vi "for_v0_v1.vi"() -> ()   [LabVIEW 2009]
panel:
  out "Numeric":dbl
  in  "Delay (ms)":dbl(slide)=101.38095238095238 min=0.0 max=2000.0 step=100.0 scale=10.0..200.0
  out "Meter":dbl(knob) scale=0.0..100.0
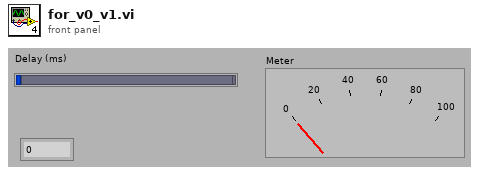
[diagram p1: front panel]
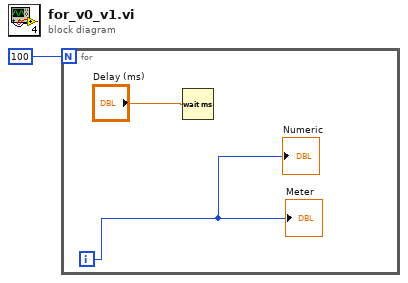
[diagram p0: block diagram]
diagram:
  n1 = for {
    N: 100 -> [_]
    i -> [w2]
    n2 = Wait (ms)(milliseconds to wait="Delay (ms)") -> ()  [unwired: 1 out]
    "Meter" <- w2
    "Numeric" <- w2
  }
